vi "SaveData.vi"(0 "Saving Actor in":refnum<class "Saving Actor.lvclass">, 1 "Path Control":path, 2 "Signal":dbl[](graph), 3 "error in (no error)":errorcluster) -> (7 "Saving Actor out":refnum<class "Saving Actor.lvclass">, 10 "error out":errorcluster)   [LabVIEW 2020, in "Saving Actor.lvlib" / "Saving Actor.lvclass"]
uses:
  Saving Actor.lvclass
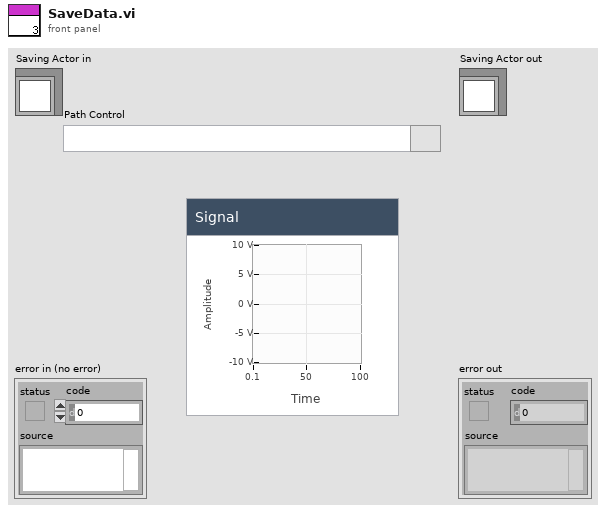
[diagram p1: front panel]
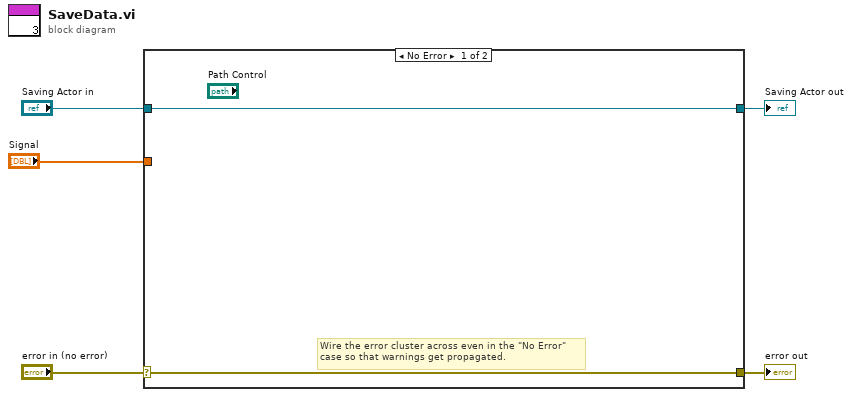
[diagram p0: block diagram]
diagram:
  n1 = case shown="No Error" "error in (no error)" {
    selector: "error in (no error)" -> [w6 w9]
    tunnel: [w6 w9] -> w4
    tunnel: [w7 w8] -> w2
    tunnel: "Saving Actor in" -> [w7 w8]
    tunnel: "Signal" -> [_ _]
    frame No Error {
      # "Wire the error cluster across even in the \"No Error\"\ncase so that warnings get propagated."
    }
    frame Error {
    }
  }
  "error out" <- w4
  "Saving Actor out" <- w2
